vi "SRDG535.contents.vi"   [LabVIEW 2014, in "SRDG535.lvlib"]
uses:
  SRDG535.lvlib
panel:
  # "This is the content vi for the SRDG535 Gate Delay Generator class"
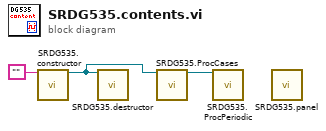
[diagram p0: block diagram]
diagram:
  n1 = call "SRDG535.constructor.vi"("name"="") -> ("i ref out"=w1:refnum<vi>)  [unwired: 16 in, 2 out]
  n2 = call "SRDG535.destructor.vi"("i ref in"=w1) -> ()  [unwired: 18 in, 1 out]
  n3 = call "SRDG535.ProcCases.vi"("i ref in"=w1) -> ("i ref out"=w3:refnum<vi>)  [unwired: 16 in, 2 out]
  n4 = call "SRDG535.ProcPeriodic.vi"("i ref in"=w3) -> ()  [unwired: 16 in, 3 out]
  n5 = call "SRDG535.panel.vi"() -> ()  [unwired: 19 in, 1 out]
